vi "CPU_Power_Spec_SGL.vi"(7 "window":u16(ring) items=["None "=0, "Hanning"=1, "Hamming"=2, "Blackman-Harris"=3, "Exact Blackman"=4, "Blackman"=5, "Flat Top"=6, "4 Term B-Harris "=7, "7 Term B-Harris"=8, "Low Sidelobe"=9, "Blackman Nuttall"=11], 11 "Signa":dbl[](array[numeric])) -> (3 "x*y":sgl[](array[numeric]))   [LabVIEW 2020]
uses:
  <vilib>/Analysis/NI_AALPro.lvlib
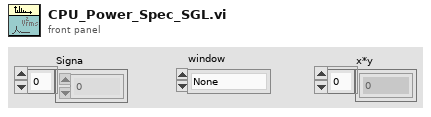
[diagram p1: front panel]
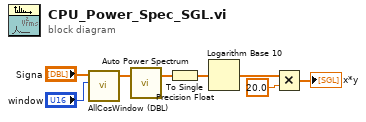
[diagram p0: block diagram]
diagram:
  n1 = call <vilib>:"AllCosWindow (DBL).vi"("window"="window", "X"="Signa") -> ("Windowed X"=w3:dbl[])  [unwired: 3 in, 1 out]
  n2 = call <vilib>:"Auto Power Spectrum.vi"("Signal (V)"=w3) -> ("Power Spectrum (V^2 rms)"=w7:dbl[])  [unwired: 1 in, 1 out]
  n3 = To Single Precision Float(number=w7) -> (single precision float=w1:sgl[])
  n4 = Logarithm Base 10(1:w1) -> (0:w6:sgl[])
  n5 = Multiply(x=w6, y=sgl 20.0 ("dt")) -> (x*y=→"x*y":sgl[])
